vi "Scale to u8.vi"(1 "Log scaling?":bool, 2 "Intensity Graph":dbl[][](graph)) -> (0 "X":u8[][](graph))   [LabVIEW 2024]
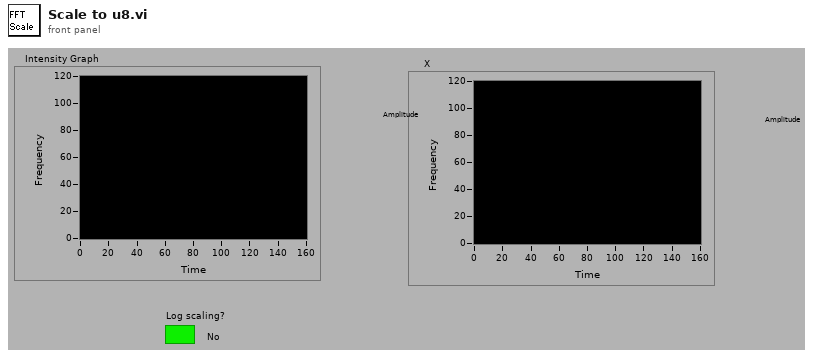
[diagram p1: front panel]
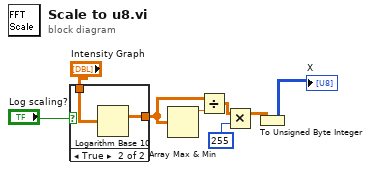
[diagram p0: block diagram]
diagram:
  n1 = case shown="True" "Log scaling?" {
    tunnel: "Intensity Graph" -> [w9 w11]
    tunnel: [w9 w10] -> w2
    frame False {
    }
    frame True {
      n2 = Logarithm Base 10(1:w11) -> (0:w10:dbl[][])
    }
  }
  n3 = Array Max & Min(array=w2) -> (max value=w3:dbl)  [unwired: 3 out]
  n4 = Divide(x=w2, y=w3) -> (x/y=w4:dbl[][])
  n5 = Multiply(x=w4, y=255) -> (x*y=w7:dbl[][])
  n6 = To Unsigned Byte Integer(number=w7) -> (unsigned 8bit integer=→"X":u8[][])
